vi "Draw point.vi"(6 "color(black)":u32(colorbox)=6618880, 9 "Coordinate":i32[](array[numeric]), 10 "rect":T1, 11 "new picture in":picture) -> (3 "new picture out":picture)   [LabVIEW 2020]
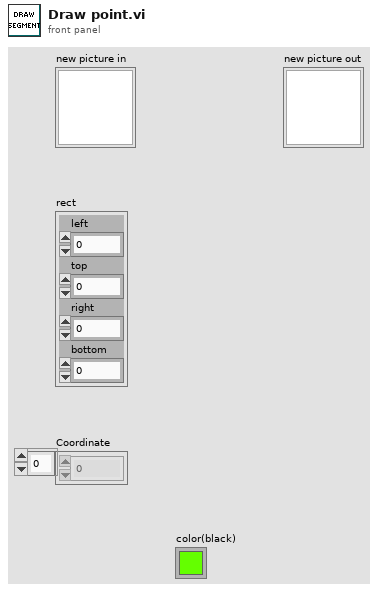
[diagram p1: front panel]
types:
  T1 = cluster{"left":i16, "top":i16, "right":i16, "bottom":i16}
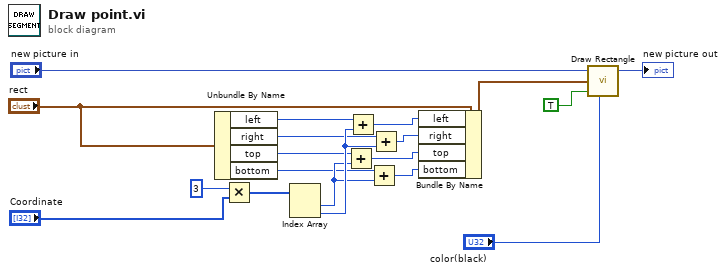
[diagram p0: block diagram]
diagram:
  n1 = Unbundle By Name("rect") -> ("left"=w12:i16, "right"=w13:i16, "top"=w9:i16, "bottom"=w10:i16)
  n2 = Multiply(x=3, y="Coordinate") -> (x*y=w8:i32[])
  n3 = Index Array(array=w8) -> (element #1=w11:i32, element #2=w14:i32)  [unwired: 2 in]
  n4 = Add(x=w9, y=w11) -> (x+y=w18:i32)
  n5 = Add(x=w12, y=w14) -> (x+y=w16:i32)
  n6 = Add(x=w10, y=w11) -> (x+y=w19:i32)
  n7 = Add(x=w13, y=w14) -> (x+y=w17:i32)
  n8 = Bundle By Name(cluster="rect", "left"=w16, "right"=w17, "top"=w18, "bottom"=w19) -> (w15:T1)
  n9 = call <vilib>:"Draw Rectangle.vi"("picture"="new picture in", "rect"=w15, "fill?(F)"=TRUE, "color(black)"="color(black)") -> ("new picture"=→"new picture out":picture)  [unwired: 5 in]
